vi "Align3DPointSetToPlane.vi"(8 "error in":errorcluster, 9 "Plane Coeffcients":T2, 11 "Point Set":T1[](array[typedef])) -> (0 "error out":errorcluster, 3 "Points Fitted to Plane":T1[](array[typedef]))   [LabVIEW 2020, in "ar.lvlib"]
uses:
  ar.lvlib
  PlaneCoeffecients.ctl
  common/Object Point (Float).ctl
  <vilib>/Analysis/baseanly.llb/Mean.vi
  <vilib>/Analysis/baseanly.llb/Mean (DBL).vi
  <vilib>/Analysis/baseanly.llb/Dot Product.vi
  <vilib>/Analysis/baseanly.llb/Real Dot Product.vi
  <vilib>/Analysis/7linalg.llb/Matrix Power.vi
  <vilib>/Analysis/7linalg.llb/Real Matrix Power.vi
  <vilib>/Analysis/_algsub.llb/Matrix Norm.vi
  <vilib>/Analysis/_algsub.llb/Real Matrix Norm.vi
  <vilib>/Analysis/7linalg.llb/SVD Decomposition.vi
  <vilib>/Analysis/7linalg.llb/Real SVD Decomposition.vi
  <vilib>/Analysis/7linalg.llb/Create Special Matrix.vi
  <vilib>/Analysis/7linalg.llb/Create Special Real Matrix.vi
  <vilib>/Analysis/coordinate.llb/Cross Product.vi
  <vilib>/Utility/error.llb/Error Cluster From Error Code.vi
  <vilib>/Analysis/Matrix/Numeric/Conversions/Array To Matrix - RA2.vi
  <vilib>/Analysis/Matrix/Numeric/Multiply/Multiply - RM,R.vi
  <vilib>/Analysis/Matrix/Numeric/Add/Add - RM,RM.vi
  <vilib>/Analysis/NI_AALBase.lvlib
  common/common.lvlib
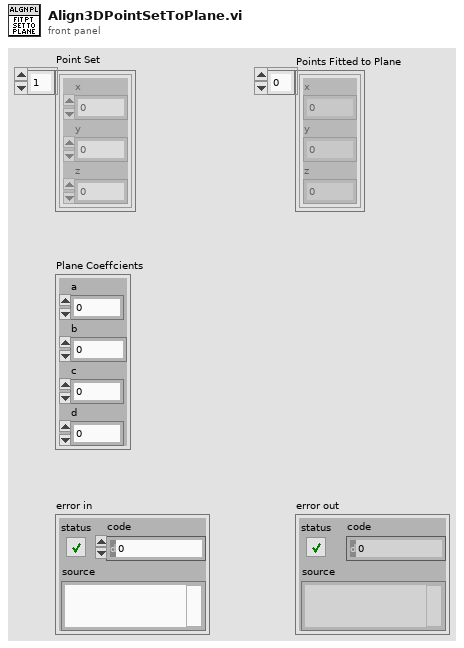
[diagram p1: front panel]
types:
  T1 = typedef "common.lvlib/Object Point (Float).ctl" = cluster{"x":dbl, "y":dbl, "z":dbl}
  T2 = typedef "ar.lvlib/PlaneCoeffecients.ctl" = cluster{"a":dbl, "b":dbl, "c":dbl, "d":dbl}
  T3 = typedef "NI_Matrix.lvlib/RealMatrix.ctl" = dbl[][]
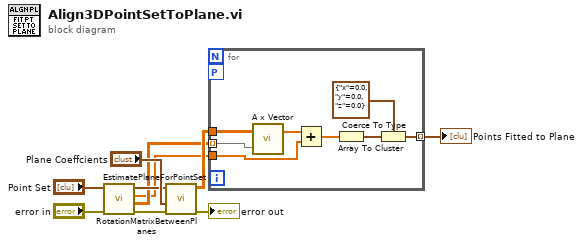
[diagram p0: block diagram]
diagram:
  n1 = call "EstimatePlaneForPointSet.vi"("error in"="error in", "Point Set"="Point Set") -> ("error out"=w7:errorcluster, "Points  Centred Around Mean Point"=w4:dbl[][], "Mean Point"=w3:dbl[], "Plane Coeffcients"=w6:T2)  [unwired: 6 in]
  n2 = call "RotationMatrixBetweenPlanes.vi"("error in"=w7, "Plane 2 Coeffcients"="Plane Coeffcients", "Plane 1 Coeffcients"=w6) -> ("error out"=→"error out":errorcluster, "Rotation Matrix"=w5:T3)  [unwired: 7 in]
  n3 = for {
    tunnel: w5 -> [w18]
    tunnel: w4 -> [w17] mode=indexing
    tunnel: w3 -> [w15]
    tunnel: [w11] -> w2 mode=indexing
    workers-P: _ -> [_]
    n4 = call <vilib>:"A x Vector.vi"("Vector"=w17, "A"=w18) -> ("A x Vector"=w16:dbl[])  [unwired: 1 out]
    n5 = Add(x=w16, y=w15) -> (x+y=w14:dbl[])
    n6 = Array To Cluster(array=w14) -> (cluster=w13:cluster{"[0]":dbl, "[1]":dbl, "[2]":dbl})
    n7 = Coerce To Type(0:w13, 1:T1 {"x"=0.0, "y"=0.0, "z"=0.0} ("Object Point")) -> (2:w11:T1)
  }
  "Points Fitted to Plane" <- w2
